vi "visible-frame-conditional-disable.vi"   [LabVIEW 2025]
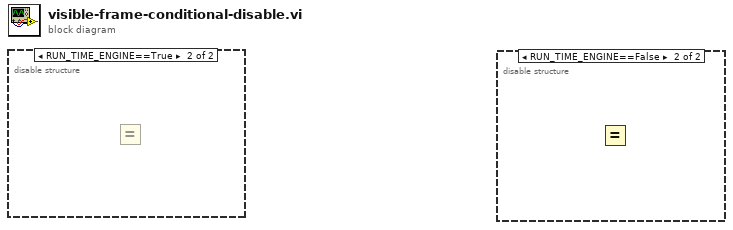
[diagram p0: block diagram]
diagram:
  n1 = disable-structure shown="RUN_TIME_ENGINE==True" {
    frame condition #0 (active) {
    }
    frame condition #1 {
      n2 = Equal?() -> ()  [unwired: 2 in, 1 out]
    }
  }
  n3 = disable-structure shown="RUN_TIME_ENGINE==False" {
    frame condition #0 {
    }
    frame condition #1 (active) {
      n4 = Equal?() -> ()  [unwired: 2 in, 1 out]
    }
  }
